vi "RIO_GetA0.vi"(0 "A[0..n]":string[](array[string])) -> (1 "A[1..n]":string[](array[string]), 2 "A[0]":string)   [LabVIEW 2012]
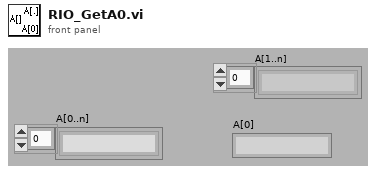
[diagram p1: front panel]
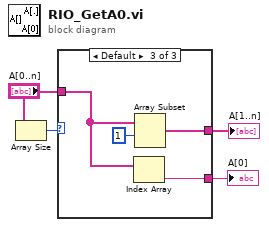
[diagram p0: block diagram]
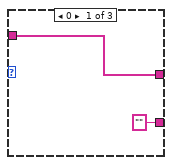
[diagram p2: hidden frame]
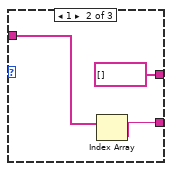
[diagram p3: hidden frame]
diagram:
  n1 = Array Size(array="A[0..n]") -> (size(s)=w2:i32)
  n2 = case shown="Default" w2 {
    tunnel: ["" w7 w13] -> w4
    tunnel: "A[0..n]" -> [w6 w8 w12]
    tunnel: [w6 string[] [] ("A[0..n]") w11] -> w3
    frame 0 {
    }
    frame 1 {
      n3 = Index Array(array=w8) -> (element=w7:string)  [unwired: 1 in]
    }
    frame Default {
      n4 = Index Array(array=w12) -> (element=w13:string)  [unwired: 1 in]
      n5 = Array Subset(array=w12, index=1) -> (w11:string[])  [unwired: 1 in]
    }
  }
  "A[0]" <- w4
  "A[1..n]" <- w3
